vi "Utility Format Pressure Compensation.vi"(8 "error in (no error)":errorcluster, 11 "Operating Pressure (PSI)":dbl) -> (0 "error out":errorcluster, 3 "Formatted Command":string)   [LabVIEW 2020, in "ChromTech Series I Drivers.lvlib"]
doc: "Formats the command to set the Pressure Compensation. The pressure given is divided by 100 and rounded to the nearest integer, so it should be provided in increments of 100 PSI to effectively change the compensation on the pump."
uses:
  <instrlib>/RxnRover/ChromtechSeriesIDriver/ChromTech Series I Drivers.lvlib
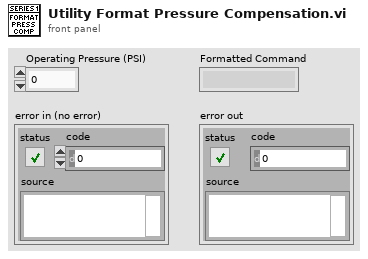
[diagram p1: front panel]
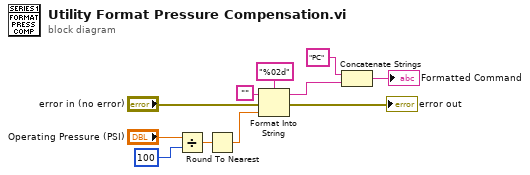
[diagram p0: block diagram]
diagram:
  n1 = Divide(x="Operating Pressure (PSI)", y=u32 100) -> (x/y=w3:dbl)
  n2 = Round To Nearest(number=w3) -> (nearest integer value=w1:dbl)
  n3 = Format Into String(format string="%02d", initial string="", error in="error in (no error)", w1) -> (resulting string=w7:string, error out=→"error out":errorcluster)
  n4 = Concatenate Strings("PC", w7) -> (→"Formatted Command":string)
